vi "电流判定.vi"(7 "Result":refnum<vi>, 9 "索引":u8, 10 "判定参数":T1, 11 "XY曲线":cluster{"X":dbl[], "Y":dbl[]}[](array[cluster])) -> (3 "OK？":bool)   [LabVIEW 2020]
panel:
  out "目标5逆向输入扭矩":dbl
  out "目标5正向输入扭矩":dbl
  out "目标 5":dbl
  out "目标4逆向输入扭矩":dbl
  out "目标4正向输入扭矩":dbl
  out "目标 4":dbl
  out "目标3逆向输入扭矩":dbl
  out "目标3正向输入扭矩":dbl
  out "目标 3":dbl
  out "目标2逆向输入扭矩":dbl
  out "目标2正向输入扭矩":dbl
  out "目标 2":dbl
  out "目标1正向输入扭矩":dbl
  out "目标1逆向输入扭矩":dbl
  out "目标 1":dbl
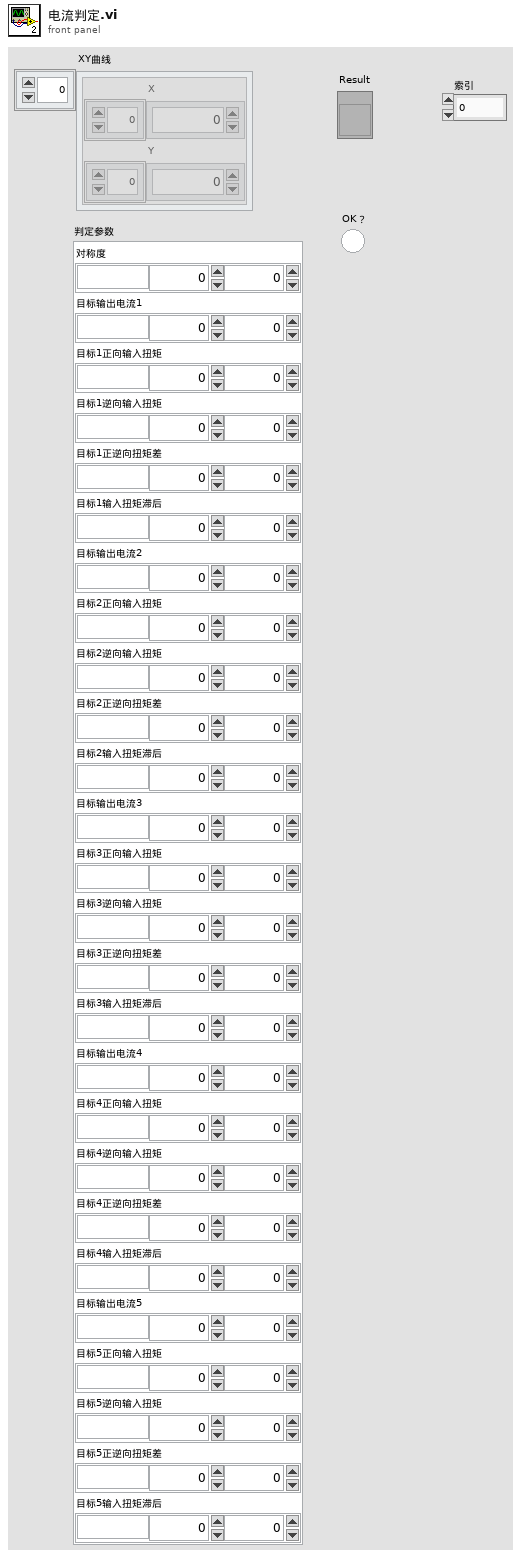
[diagram p1: front panel]
types:
  T1 = cluster{"对称度":cluster{"单位":string, "下限":dbl, "上限":dbl}, "目标输出电流1":cluster{"单位":string, "下限":dbl, "上限":dbl}, "目标1正向输入扭矩":cluster{"单位":string, "下限":dbl, "上限":dbl}, "目标1逆向输入扭矩":cluster{"单位":string, "下限":dbl, "上限":dbl}, "目标1正逆向扭矩差":cluster{"单位":string, "下限":dbl, "上限":dbl}, "目标1输入扭矩滞后":cluster{"单位":string, "下限":dbl, "上限":dbl}, "目标输出电流2":cluster{"单位":string, "下限":dbl, "上限":dbl}, "目标2正向输入扭矩":cluster{"单位":string, "下限":dbl, "上限":dbl}, "目标2逆向输入扭矩":cluster{"单位":string, "下限":dbl, "上限":dbl}, "目标2正逆向扭矩差":cluster{"单位":string, "下限":dbl, "上限":dbl}, "目标2输入扭矩滞后":cluster{"单位":string, "下限":dbl, "上限":dbl}, "目标输出电流3":cluster{"单位":string, "下限":dbl, "上限":dbl}, "目标3正向输入扭矩":cluster{"单位":string, "下限":dbl, "上限":dbl}, "目标3逆向输入扭矩":cluster{"单位":string, "下限":dbl, "上限":dbl}, "目标3正逆向扭矩差":cluster{"单位":string, "下限":dbl, "上限":dbl}, "目标3输入扭矩滞后":cluster{"单位":string, "下限":dbl, "上限":dbl}, "目标输出电流4":cluster{"单位":string, "下限":dbl, "上限":dbl}, "目标4正向输入扭矩":cluster{"单位":string, "下限":dbl, "上限":dbl}, "目标4逆向输入扭矩":cluster{"单位":string, "下限":dbl, "上限":dbl}, "目标4正逆向扭矩差":cluster{"单位":string, "下限":dbl, "上限":dbl}, "目标4输入扭矩滞后":cluster{"单位":string, "下限":dbl, "上限":dbl}, "目标输出电流5":cluster{"单位":string, "下限":dbl, "上限":dbl}, "目标5正向输入扭矩":cluster{"单位":string, "下限":dbl, "上限":dbl}, "目标5逆向输入扭矩":cluster{"单位":string, "下限":dbl, "上限":dbl}, "目标5正逆向扭矩差":cluster{"单位":string, "下限":dbl, "上限":dbl}, "目标5输入扭矩滞后":cluster{"单位":string, "下限":dbl, "上限":dbl}}
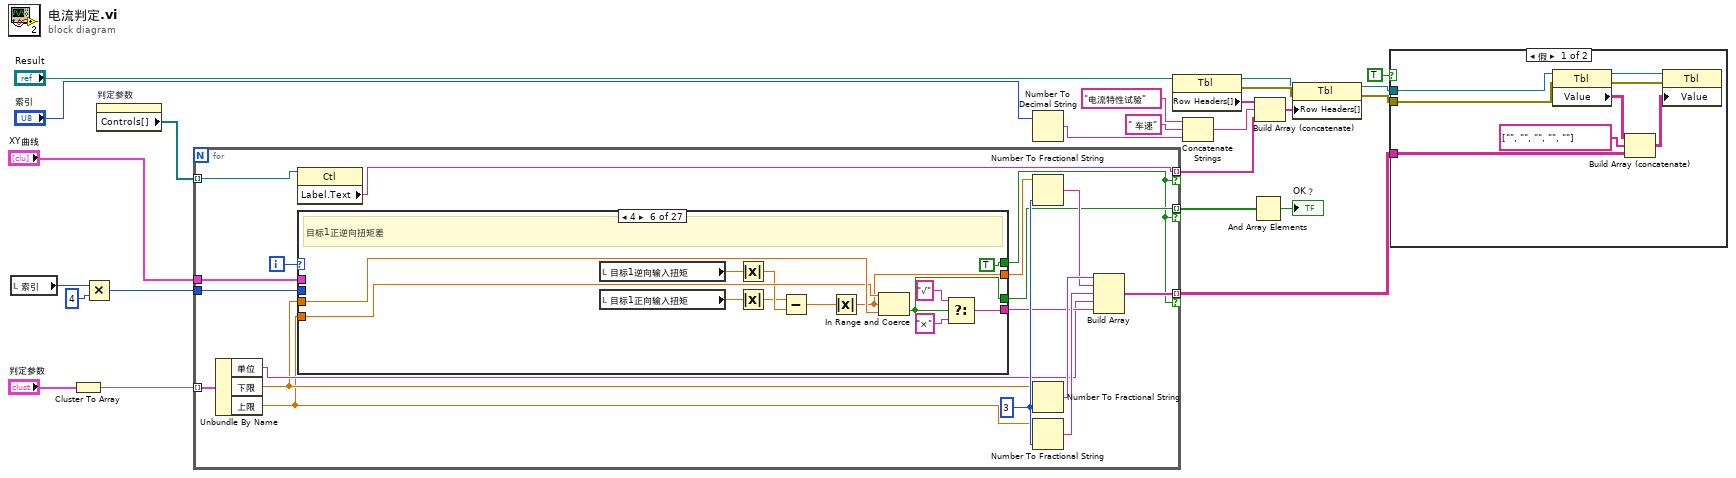
[diagram p0: block diagram]
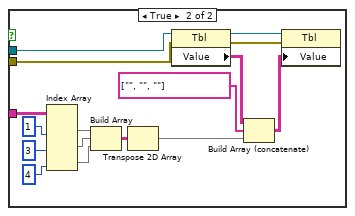
[diagram p2: hidden frame]
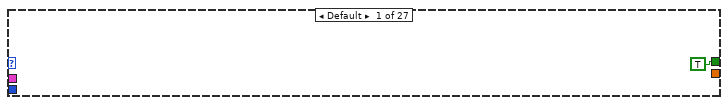
[diagram p3: hidden frame]
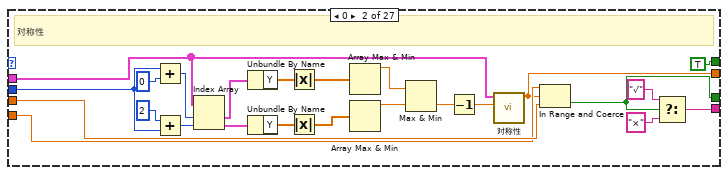
[diagram p4: hidden frame]
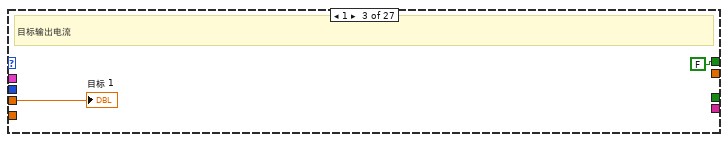
[diagram p5: hidden frame]
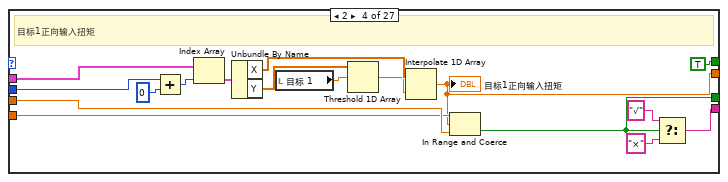
[diagram p6: hidden frame]
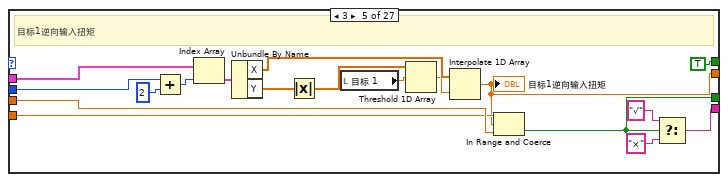
[diagram p7: hidden frame]
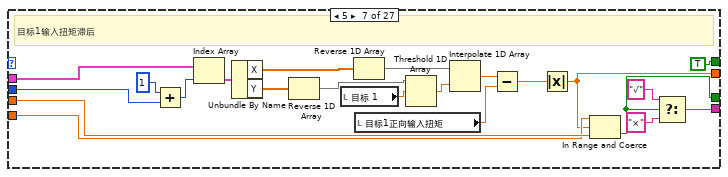
[diagram p8: hidden frame]
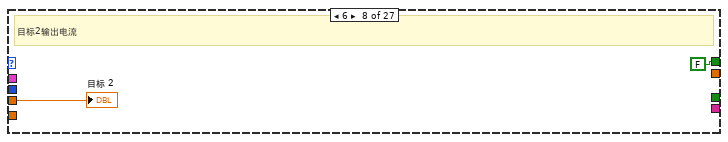
[diagram p9: hidden frame]
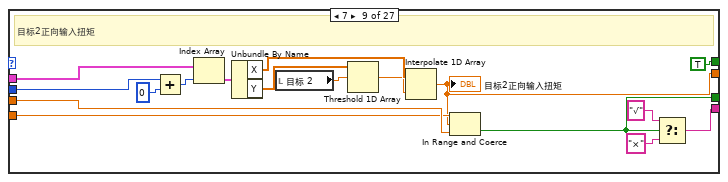
[diagram p10: hidden frame]
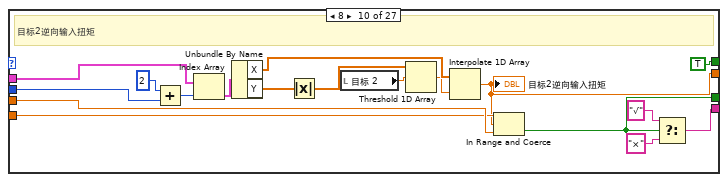
[diagram p11: hidden frame]
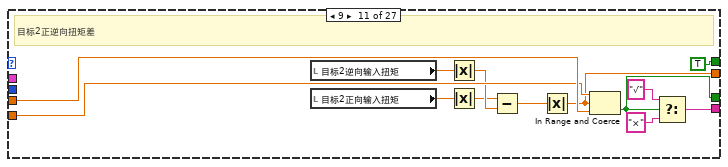
[diagram p12: hidden frame]
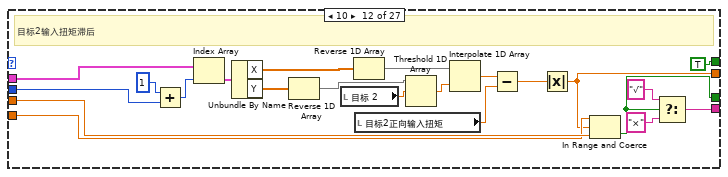
[diagram p13: hidden frame]
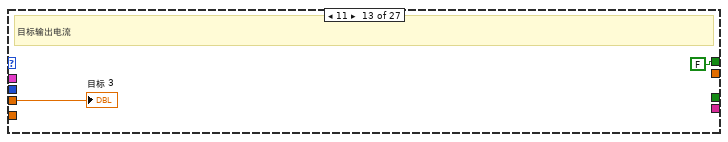
[diagram p14: hidden frame]
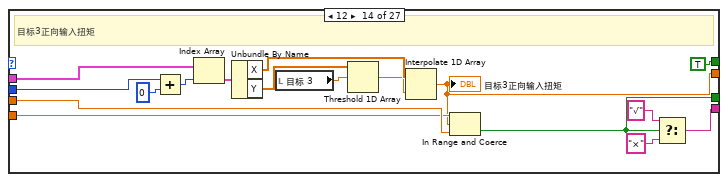
[diagram p15: hidden frame]
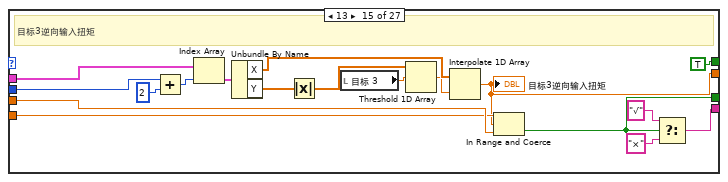
[diagram p16: hidden frame]
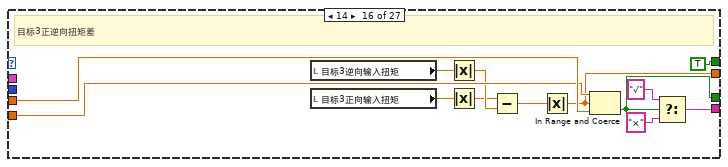
[diagram p17: hidden frame]
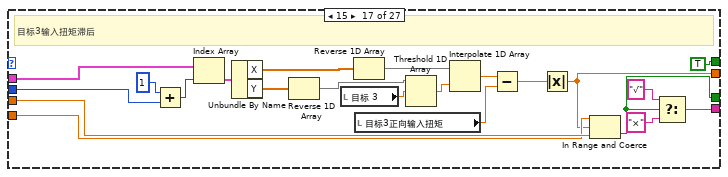
[diagram p18: hidden frame]
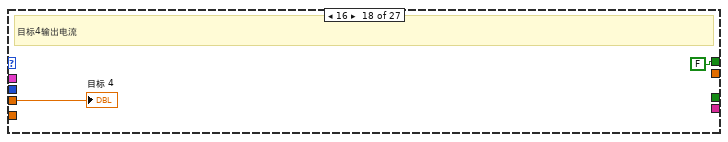
[diagram p19: hidden frame]
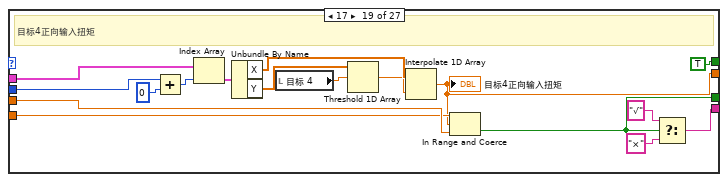
[diagram p20: hidden frame]
diagram:
  n1 = local read "索引"() -> (w3:u8)
  n2 = Cluster To Array(cluster="判定参数") -> (array=w24:cluster{"单位":string, "下限":dbl, "上限":dbl}[])
  n3 = Multiply(x=w3, y=u8 4) -> (x*y=w1:u8)
  n4 = property on="判定参数" class="Clust (严格)"() -> ("Controls[]"=w10:refnum<vi>[])  [unwired: 2 in, 2 out]
  n5 = for {
    tunnel: w24 -> [w42] mode=indexing
    tunnel: w10 -> [w40] mode=indexing
    tunnel: "XY曲线" -> [w38]
    tunnel: [w32] -> w22 mode=indexing if=w26
    tunnel: [w28] -> w12 mode=indexing if=w26
    tunnel: [w27] -> w15 mode=indexing if=w26
    tunnel: w1 -> [w25]
    i -> [w41]
    w37 = i16 3 ("精度(6)")
    n6 = Unbundle By Name(w42) -> ("单位"=w31:string, "下限"=w30:dbl, "上限"=w29:dbl)
    n7 = property class="Ctl"(reference=w40) -> ("Label.Text"=w27:string)  [unwired: 1 in, 2 out]
    n8 = case shown="4" w41 {
      tunnel: [_ w52 _ w72 w91 w107 w121 _ w144 w163 w179 w193 _ w216 w235 w251 w265 _ w288 w307 w323 w337 _ w360 w379 w395 w409] -> w39
      tunnel: w38 -> [_ w56 _ w79 w97 _ w133 _ w151 w169 _ w205 _ w223 w241 _ w277 _ w295 w313 _ w349 _ w367 w385 _ w421]
      tunnel: [_ w61 _ w84 w102 w115 w122 _ w156 w174 w187 w194 _ w228 w246 w259 w266 _ w300 w318 w331 w338 _ w372 w390 w403 w410] -> w33
      tunnel: [_ w60 _ w83 w101 w114 w123 _ w155 w173 w186 w195 _ w227 w245 w258 w267 _ w299 w317 w330 w339 _ w371 w389 w402 w411] -> w32
      tunnel: w30 -> [_ w59 w68 w82 w100 w113 w127 w140 w154 w172 w185 w199 w212 w226 w244 w257 w271 w284 w298 w316 w329 w343 w356 w370 w388 w401 w415]
      tunnel: w29 -> [_ w58 _ w81 w99 w112 w126 _ w153 w171 w184 w198 _ w225 w243 w256 w270 _ w297 w315 w328 w342 _ w369 w387 w400 w414]
      tunnel: [TRUE TRUE FALSE TRUE TRUE TRUE TRUE FALSE TRUE TRUE TRUE TRUE FALSE TRUE TRUE TRUE TRUE FALSE TRUE TRUE TRUE TRUE FALSE TRUE TRUE TRUE TRUE] -> w26
      tunnel: w25 -> [_ w44 _ w70 w87 _ w118 _ w142 w159 _ w190 _ w214 w231 _ w262 _ w286 w303 _ w334 _ w358 w375 _ w406]
      frame Default {
      }
      frame 0 {
        # "对称性"
        n9 = Add(x=w44, y=0 ("索引")) -> (x+y=w46:i32)
        n10 = Add(x=2 ("索引"), y=w44) -> (x+y=w45:i32)
        n11 = Index Array(array=w56, index #1=w46, index #2=w45) -> (element #1=w65:cluster{"X":dbl[], "Y":dbl[]}, element #2=w64:cluster{"X":dbl[], "Y":dbl[]})
        n12 = Unbundle By Name(w65) -> ("Y"=w55:dbl[])
        n13 = Unbundle By Name(w64) -> ("Y"=w54:dbl[])
        n14 = Absolute Value(x=w55) -> (abs(x)=w51:dbl[])
        n15 = Absolute Value(x=w54) -> (abs(x)=w50:dbl[])
        n16 = Array Max & Min(array=w51) -> (max value=w49:dbl)  [unwired: 3 out]
        n17 = Array Max & Min(array=w50) -> (max value=w48:dbl)  [unwired: 3 out]
        n18 = Max & Min(x=w49, y=w48) -> (min(x,y)=w53:dbl)  [unwired: 1 out]
        n19 = Decrement(x=w53) -> (x-1=w47:dbl)
        n20 = call "对称性.vi"("定点"=w47, "XY图"=w56) -> ("对称性"=w52:dbl)  [unwired: 9 in]
        n21 = In Range and Coerce(upper limit=w58, x=w52, lower limit=w59) -> (In Range?=w60:bool)  [unwired: 1 out]
        n22 = Select(t="√", s=w60, f="×") -> (s? t:f=w61:string)
      }
      frame 1 {
        # "目标输出电流"
        "目标 1" <- w68
      }
      frame 2 {
        # "目标1正向输入扭矩"
        n23 = Add(x=w70, y=0 ("索引")) -> (x+y=w71:i32)
        n24 = Index Array(array=w79, index=w71) -> (element=w78:cluster{"X":dbl[], "Y":dbl[]})
        n25 = Unbundle By Name(w78) -> ("X"=w75:dbl[], "Y"=w77:dbl[])
        n26 = local read "目标 1"() -> (w76:dbl)
        n27 = Threshold 1D Array(2:w76, 3:w77) -> (0:w74:dbl)  [unwired: 1 in]
        n28 = Interpolate 1D Array(1:w74, 2:w75) -> (0:w72:dbl)
        "目标1正向输入扭矩" <- w72
        n29 = In Range and Coerce(upper limit=w81, x=w72, lower limit=w82) -> (In Range?=w83:bool)  [unwired: 1 out]
        n30 = Select(t="√", s=w83, f="×") -> (s? t:f=w84:string)
      }
      frame 3 {
        # "目标1逆向输入扭矩"
        n31 = Add(x=w87, y=2 ("索引")) -> (x+y=w88:i32)
        n32 = Index Array(array=w97, index=w88) -> (element=w96:cluster{"X":dbl[], "Y":dbl[]})
        n33 = Unbundle By Name(w96) -> ("X"=w93:dbl[], "Y"=w95:dbl[])
        n34 = Absolute Value(x=w95) -> (abs(x)=w89:dbl[])
        n35 = local read "目标 1"() -> (w94:dbl)
        n36 = Threshold 1D Array(2:w94, 3:w89) -> (0:w92:dbl)  [unwired: 1 in]
        n37 = Interpolate 1D Array(1:w92, 2:w93) -> (0:w91:dbl)
        "目标1逆向输入扭矩" <- w91
        n38 = In Range and Coerce(upper limit=w99, x=w91, lower limit=w100) -> (In Range?=w101:bool)  [unwired: 1 out]
        n39 = Select(t="√", s=w101, f="×") -> (s? t:f=w102:string)
      }
      frame 4 {
        # "目标1正逆向扭矩差"
        n40 = local read "目标1逆向输入扭矩"() -> (w109:dbl)
        n41 = local read "目标1正向输入扭矩"() -> (w110:dbl)
        n42 = Absolute Value(x=w109) -> (abs(x)=w106:dbl)
        n43 = Absolute Value(x=w110) -> (abs(x)=w105:dbl)
        n44 = Subtract(x=w105, y=w106) -> (x-y=w108:dbl)
        n45 = Absolute Value(x=w108) -> (abs(x)=w107:dbl)
        n46 = In Range and Coerce(upper limit=w112, x=w107, lower limit=w113) -> (In Range?=w114:bool)  [unwired: 1 out]
        n47 = Select(t="√", s=w114, f="×") -> (s? t:f=w115:string)
      }
      frame 5 {
        # "目标1输入扭矩滞后"
        n48 = Add(x=1 ("索引"), y=w118) -> (x+y=w119:i32)
        n49 = Index Array(array=w133, index=w119) -> (element=w139:cluster{"X":dbl[], "Y":dbl[]})
        n50 = Unbundle By Name(w139) -> ("X"=w136:dbl[], "Y"=w138:dbl[])
        n51 = Reverse 1D Array(array=w138) -> (reversed array=w132:dbl[])
        n52 = local read "目标 1"() -> (w137:dbl)
        n53 = Reverse 1D Array(array=w136) -> (reversed array=w131:dbl[])
        n54 = local read "目标1正向输入扭矩"() -> (w129:dbl)
        n55 = Threshold 1D Array(2:w137, 3:w132) -> (0:w135:dbl)  [unwired: 1 in]
        n56 = Interpolate 1D Array(1:w135, 2:w131) -> (0:w130:dbl)
        n57 = Subtract(x=w130, y=w129) -> (x-y=w128:dbl)
        n58 = Absolute Value(x=w128) -> (abs(x)=w121:dbl)
        n59 = In Range and Coerce(upper limit=w126, x=w121, lower limit=w127) -> (In Range?=w123:bool)  [unwired: 1 out]
        n60 = Select(t="√", s=w123, f="×") -> (s? t:f=w122:string)
      }
      frame 6 {
        # "目标2输出电流"
        "目标 2" <- w140
      }
      frame 7 {
        # "目标2正向输入扭矩"
        n61 = Add(x=w142, y=0 ("索引")) -> (x+y=w143:i32)
        n62 = Index Array(array=w151, index=w143) -> (element=w150:cluster{"X":dbl[], "Y":dbl[]})
        n63 = Unbundle By Name(w150) -> ("X"=w147:dbl[], "Y"=w149:dbl[])
        n64 = local read "目标 2"() -> (w148:dbl)
        n65 = Threshold 1D Array(2:w148, 3:w149) -> (0:w146:dbl)  [unwired: 1 in]
        n66 = Interpolate 1D Array(1:w146, 2:w147) -> (0:w144:dbl)
        "目标2正向输入扭矩" <- w144
        n67 = In Range and Coerce(upper limit=w153, x=w144, lower limit=w154) -> (In Range?=w155:bool)  [unwired: 1 out]
        n68 = Select(t="√", s=w155, f="×") -> (s? t:f=w156:string)
      }
      frame 8 {
        # "目标2逆向输入扭矩"
        n69 = Add(x=2 ("索引"), y=w159) -> (x+y=w160:i32)
        n70 = Index Array(array=w169, index=w160) -> (element=w168:cluster{"X":dbl[], "Y":dbl[]})
        n71 = Unbundle By Name(w168) -> ("X"=w165:dbl[], "Y"=w167:dbl[])
        n72 = Absolute Value(x=w167) -> (abs(x)=w161:dbl[])
        n73 = local read "目标 2"() -> (w166:dbl)
        n74 = Threshold 1D Array(2:w166, 3:w161) -> (0:w164:dbl)  [unwired: 1 in]
        n75 = Interpolate 1D Array(1:w164, 2:w165) -> (0:w163:dbl)
        "目标2逆向输入扭矩" <- w163
        n76 = In Range and Coerce(upper limit=w171, x=w163, lower limit=w172) -> (In Range?=w173:bool)  [unwired: 1 out]
        n77 = Select(t="√", s=w173, f="×") -> (s? t:f=w174:string)
      }
      frame 9 {
        # "目标2正逆向扭矩差"
        n78 = local read "目标2逆向输入扭矩"() -> (w181:dbl)
        n79 = local read "目标2正向输入扭矩"() -> (w182:dbl)
        n80 = Absolute Value(x=w181) -> (abs(x)=w178:dbl)
        n81 = Absolute Value(x=w182) -> (abs(x)=w177:dbl)
        n82 = Subtract(x=w177, y=w178) -> (x-y=w180:dbl)
        n83 = Absolute Value(x=w180) -> (abs(x)=w179:dbl)
        n84 = In Range and Coerce(upper limit=w184, x=w179, lower limit=w185) -> (In Range?=w186:bool)  [unwired: 1 out]
        n85 = Select(t="√", s=w186, f="×") -> (s? t:f=w187:string)
      }
      frame 10 {
        # "目标2输入扭矩滞后"
        n86 = Add(x=1 ("索引"), y=w190) -> (x+y=w191:i32)
        n87 = Index Array(array=w205, index=w191) -> (element=w211:cluster{"X":dbl[], "Y":dbl[]})
        n88 = Unbundle By Name(w211) -> ("X"=w208:dbl[], "Y"=w210:dbl[])
        n89 = Reverse 1D Array(array=w210) -> (reversed array=w204:dbl[])
        n90 = local read "目标 2"() -> (w209:dbl)
        n91 = Reverse 1D Array(array=w208) -> (reversed array=w203:dbl[])
        n92 = local read "目标2正向输入扭矩"() -> (w201:dbl)
        n93 = Threshold 1D Array(2:w209, 3:w204) -> (0:w207:dbl)  [unwired: 1 in]
        n94 = Interpolate 1D Array(1:w207, 2:w203) -> (0:w202:dbl)
        n95 = Subtract(x=w202, y=w201) -> (x-y=w200:dbl)
        n96 = Absolute Value(x=w200) -> (abs(x)=w193:dbl)
        n97 = In Range and Coerce(upper limit=w198, x=w193, lower limit=w199) -> (In Range?=w195:bool)  [unwired: 1 out]
        n98 = Select(t="√", s=w195, f="×") -> (s? t:f=w194:string)
      }
      frame 11 {
        # "目标输出电流"
        "目标 3" <- w212
      }
      frame 12 {
        # "目标3正向输入扭矩"
        n99 = Add(x=w214, y=0 ("索引")) -> (x+y=w215:i32)
        n100 = Index Array(array=w223, index=w215) -> (element=w222:cluster{"X":dbl[], "Y":dbl[]})
        n101 = Unbundle By Name(w222) -> ("X"=w219:dbl[], "Y"=w221:dbl[])
        n102 = local read "目标 3"() -> (w220:dbl)
        n103 = Threshold 1D Array(2:w220, 3:w221) -> (0:w218:dbl)  [unwired: 1 in]
        n104 = Interpolate 1D Array(1:w218, 2:w219) -> (0:w216:dbl)
        "目标3正向输入扭矩" <- w216
        n105 = In Range and Coerce(upper limit=w225, x=w216, lower limit=w226) -> (In Range?=w227:bool)  [unwired: 1 out]
        n106 = Select(t="√", s=w227, f="×") -> (s? t:f=w228:string)
      }
      frame 13 {
        # "目标3逆向输入扭矩"
        n107 = Add(x=w231, y=2 ("索引")) -> (x+y=w232:i32)
        n108 = Index Array(array=w241, index=w232) -> (element=w240:cluster{"X":dbl[], "Y":dbl[]})
        n109 = Unbundle By Name(w240) -> ("X"=w237:dbl[], "Y"=w239:dbl[])
        n110 = Absolute Value(x=w239) -> (abs(x)=w233:dbl[])
        n111 = local read "目标 3"() -> (w238:dbl)
        n112 = Threshold 1D Array(2:w238, 3:w233) -> (0:w236:dbl)  [unwired: 1 in]
        n113 = Interpolate 1D Array(1:w236, 2:w237) -> (0:w235:dbl)
        "目标3逆向输入扭矩" <- w235
        n114 = In Range and Coerce(upper limit=w243, x=w235, lower limit=w244) -> (In Range?=w245:bool)  [unwired: 1 out]
        n115 = Select(t="√", s=w245, f="×") -> (s? t:f=w246:string)
      }
      frame 14 {
        # "目标3正逆向扭矩差"
        n116 = local read "目标3逆向输入扭矩"() -> (w253:dbl)
        n117 = local read "目标3正向输入扭矩"() -> (w254:dbl)
        n118 = Absolute Value(x=w253) -> (abs(x)=w250:dbl)
        n119 = Absolute Value(x=w254) -> (abs(x)=w249:dbl)
        n120 = Subtract(x=w249, y=w250) -> (x-y=w252:dbl)
        n121 = Absolute Value(x=w252) -> (abs(x)=w251:dbl)
        n122 = In Range and Coerce(upper limit=w256, x=w251, lower limit=w257) -> (In Range?=w258:bool)  [unwired: 1 out]
        n123 = Select(t="√", s=w258, f="×") -> (s? t:f=w259:string)
      }
      frame 15 {
        # "目标3输入扭矩滞后"
        n124 = Add(x=1 ("索引"), y=w262) -> (x+y=w263:i32)
        n125 = Index Array(array=w277, index=w263) -> (element=w283:cluster{"X":dbl[], "Y":dbl[]})
        n126 = Unbundle By Name(w283) -> ("X"=w280:dbl[], "Y"=w282:dbl[])
        n127 = Reverse 1D Array(array=w282) -> (reversed array=w276:dbl[])
        n128 = local read "目标 3"() -> (w281:dbl)
        n129 = Reverse 1D Array(array=w280) -> (reversed array=w275:dbl[])
        n130 = local read "目标3正向输入扭矩"() -> (w273:dbl)
        n131 = Threshold 1D Array(2:w281, 3:w276) -> (0:w279:dbl)  [unwired: 1 in]
        n132 = Interpolate 1D Array(1:w279, 2:w275) -> (0:w274:dbl)
        n133 = Subtract(x=w274, y=w273) -> (x-y=w272:dbl)
        n134 = Absolute Value(x=w272) -> (abs(x)=w265:dbl)
        n135 = In Range and Coerce(upper limit=w270, x=w265, lower limit=w271) -> (In Range?=w267:bool)  [unwired: 1 out]
        n136 = Select(t="√", s=w267, f="×") -> (s? t:f=w266:string)
      }
      frame 16 {
        # "目标4输出电流"
        "目标 4" <- w284
      }
      frame 17 {
        # "目标4正向输入扭矩"
        n137 = Add(x=w286, y=0 ("索引")) -> (x+y=w287:i32)
        n138 = Index Array(array=w295, index=w287) -> (element=w294:cluster{"X":dbl[], "Y":dbl[]})
        n139 = Unbundle By Name(w294) -> ("X"=w291:dbl[], "Y"=w293:dbl[])
        n140 = local read "目标 4"() -> (w292:dbl)
        n141 = Threshold 1D Array(2:w292, 3:w293) -> (0:w290:dbl)  [unwired: 1 in]
        n142 = Interpolate 1D Array(1:w290, 2:w291) -> (0:w288:dbl)
        "目标4正向输入扭矩" <- w288
        n143 = In Range and Coerce(upper limit=w297, x=w288, lower limit=w298) -> (In Range?=w299:bool)  [unwired: 1 out]
        n144 = Select(t="√", s=w299, f="×") -> (s? t:f=w300:string)
      }
      frame 18 {
        # "目标4逆向输入扭矩"
        n145 = Add(x=w303, y=2 ("索引")) -> (x+y=w304:i32)
        n146 = Index Array(array=w313, index=w304) -> (element=w312:cluster{"X":dbl[], "Y":dbl[]})
        n147 = Unbundle By Name(w312) -> ("X"=w309:dbl[], "Y"=w311:dbl[])
        n148 = Absolute Value(x=w311) -> (abs(x)=w305:dbl[])
        n149 = local read "目标 4"() -> (w310:dbl)
        n150 = Threshold 1D Array(2:w310, 3:w305) -> (0:w308:dbl)  [unwired: 1 in]
        n151 = Interpolate 1D Array(1:w308, 2:w309) -> (0:w307:dbl)
        "目标4逆向输入扭矩" <- w307
        n152 = In Range and Coerce(upper limit=w315, x=w307, lower limit=w316) -> (In Range?=w317:bool)  [unwired: 1 out]
        n153 = Select(t="√", s=w317, f="×") -> (s? t:f=w318:string)
      }
      frame 19 {
        # "目标4正逆向扭矩差"
        n154 = local read "目标4逆向输入扭矩"() -> (w325:dbl)
        n155 = local read "目标4正向输入扭矩"() -> (w326:dbl)
        n156 = Absolute Value(x=w325) -> (abs(x)=w322:dbl)
        n157 = Absolute Value(x=w326) -> (abs(x)=w321:dbl)
        n158 = Subtract(x=w321, y=w322) -> (x-y=w324:dbl)
        n159 = Absolute Value(x=w324) -> (abs(x)=w323:dbl)
        n160 = In Range and Coerce(upper limit=w328, x=w323, lower limit=w329) -> (In Range?=w330:bool)  [unwired: 1 out]
        n161 = Select(t="√", s=w330, f="×") -> (s? t:f=w331:string)
      }
      frame 20 {
        # "目标4输入扭矩滞后"
        n162 = Add(x=w334, y=1 ("索引")) -> (x+y=w335:i32)
        n163 = Index Array(array=w349, index=w335) -> (element=w355:cluster{"X":dbl[], "Y":dbl[]})
        n164 = Unbundle By Name(w355) -> ("X"=w352:dbl[], "Y"=w354:dbl[])
        n165 = Reverse 1D Array(array=w354) -> (reversed array=w348:dbl[])
        n166 = local read "目标 4"() -> (w353:dbl)
        n167 = Reverse 1D Array(array=w352) -> (reversed array=w347:dbl[])
        n168 = local read "目标4正向输入扭矩"() -> (w345:dbl)
        n169 = Threshold 1D Array(2:w353, 3:w348) -> (0:w351:dbl)  [unwired: 1 in]
        n170 = Interpolate 1D Array(1:w351, 2:w347) -> (0:w346:dbl)
        n171 = Subtract(x=w346, y=w345) -> (x-y=w344:dbl)
        n172 = Absolute Value(x=w344) -> (abs(x)=w337:dbl)
        n173 = In Range and Coerce(upper limit=w342, x=w337, lower limit=w343) -> (In Range?=w339:bool)  [unwired: 1 out]
        n174 = Select(t="√", s=w339, f="×") -> (s? t:f=w338:string)
      }
      frame 21 {
        # "目标5输出电流"
        "目标 5" <- w356
      }
      frame 22 {
        # "目标5正向输入扭矩"
        n175 = Add(x=0 ("索引"), y=w358) -> (x+y=w359:i32)
        n176 = Index Array(array=w367, index=w359) -> (element=w366:cluster{"X":dbl[], "Y":dbl[]})
        n177 = Unbundle By Name(w366) -> ("X"=w363:dbl[], "Y"=w365:dbl[])
        n178 = local read "目标 5"() -> (w364:dbl)
        n179 = Threshold 1D Array(2:w364, 3:w365) -> (0:w362:dbl)  [unwired: 1 in]
        n180 = Interpolate 1D Array(1:w362, 2:w363) -> (0:w360:dbl)
        "目标5正向输入扭矩" <- w360
        n181 = In Range and Coerce(upper limit=w369, x=w360, lower limit=w370) -> (In Range?=w371:bool)  [unwired: 1 out]
        n182 = Select(t="√", s=w371, f="×") -> (s? t:f=w372:string)
      }
      frame 23 {
        # "目标5逆向输入扭矩"
        n183 = Add(x=2 ("索引"), y=w375) -> (x+y=w376:i32)
        n184 = Index Array(array=w385, index=w376) -> (element=w384:cluster{"X":dbl[], "Y":dbl[]})
        n185 = Unbundle By Name(w384) -> ("X"=w381:dbl[], "Y"=w383:dbl[])
        n186 = Absolute Value(x=w383) -> (abs(x)=w377:dbl[])
        n187 = local read "目标 5"() -> (w382:dbl)
        n188 = Threshold 1D Array(2:w382, 3:w377) -> (0:w380:dbl)  [unwired: 1 in]
        n189 = Interpolate 1D Array(1:w380, 2:w381) -> (0:w379:dbl)
        "目标5逆向输入扭矩" <- w379
        n190 = In Range and Coerce(upper limit=w387, x=w379, lower limit=w388) -> (In Range?=w389:bool)  [unwired: 1 out]
        n191 = Select(t="√", s=w389, f="×") -> (s? t:f=w390:string)
      }
      frame 24 {
        # "目标5正逆向扭矩差"
        n192 = local read "目标5逆向输入扭矩"() -> (w397:dbl)
        n193 = local read "目标5正向输入扭矩"() -> (w398:dbl)
        n194 = Absolute Value(x=w397) -> (abs(x)=w394:dbl)
        n195 = Absolute Value(x=w398) -> (abs(x)=w393:dbl)
        n196 = Subtract(x=w393, y=w394) -> (x-y=w396:dbl)
        n197 = Absolute Value(x=w396) -> (abs(x)=w395:dbl)
        n198 = In Range and Coerce(upper limit=w400, x=w395, lower limit=w401) -> (In Range?=w402:bool)  [unwired: 1 out]
        n199 = Select(t="√", s=w402, f="×") -> (s? t:f=w403:string)
      }
      frame 25 {
        # "目标5输入扭矩滞后"
        n200 = Add(x=1 ("索引"), y=w406) -> (x+y=w407:i32)
        n201 = Index Array(array=w421, index=w407) -> (element=w427:cluster{"X":dbl[], "Y":dbl[]})
        n202 = Unbundle By Name(w427) -> ("X"=w424:dbl[], "Y"=w426:dbl[])
        n203 = Reverse 1D Array(array=w426) -> (reversed array=w420:dbl[])
        n204 = local read "目标 5"() -> (w425:dbl)
        n205 = Reverse 1D Array(array=w424) -> (reversed array=w419:dbl[])
        n206 = local read "目标5正向输入扭矩"() -> (w417:dbl)
        n207 = Threshold 1D Array(2:w425, 3:w420) -> (0:w423:dbl)  [unwired: 1 in]
        n208 = Interpolate 1D Array(1:w423, 2:w419) -> (0:w418:dbl)
        n209 = Subtract(x=w418, y=w417) -> (x-y=w416:dbl)
        n210 = Absolute Value(x=w416) -> (abs(x)=w409:dbl)
        n211 = In Range and Coerce(upper limit=w414, x=w409, lower limit=w415) -> (In Range?=w411:bool)  [unwired: 1 out]
        n212 = Select(t="√", s=w411, f="×") -> (s? t:f=w410:string)
      }
    }
    n213 = Number To Fractional String(number=w39, precision (6)=w37) -> (F-format string=w35:string)  [unwired: 2 in]
    n214 = Number To Fractional String(number=w30, precision (6)=w37) -> (F-format string=w36:string)  [unwired: 2 in]
    n215 = Number To Fractional String(number=w29, precision (6)=w37) -> (F-format string=w34:string)  [unwired: 2 in]
    n216 = Build Array(w36, w35, w34, w31, w33) -> (w28:string[])
  }
  n217 = Number To Decimal String(number="索引") -> (decimal integer string=w7:string)  [unwired: 1 in]
  n218 = property class="Tbl"(reference="Result") -> (reference out=w17:refnum<vi>, error out=w20:errorcluster, "Row Headers[]"=w13:string[])  [unwired: 1 in]
  n219 = Concatenate Strings("电流特性试验" ("Label.Text"), " 车速" ("字符串"), w7) -> (w4:string)
  n220 = And Array Elements(Boolean array=w22) -> (logical AND=→"OK？":bool)
  n221 = Build Array (concatenate)(w13, w4, w15) -> (w16:string[])
  n222 = property class="Tbl"(reference=w17, error in=w20, "Row Headers[]"=w16) -> (reference out=w18:refnum<vi>, error out=w19:errorcluster)
  n223 = case shown="假" TRUE {
    tunnel: w19 -> [w433 w449]
    tunnel: w18 -> [w430 w446]
    tunnel: w12 -> [w429 w437]
    frame False {
      n224 = property class="Tbl"(reference=w430, error in=w433) -> (reference out=w431:refnum<vi>, error out=w432:errorcluster, "Value"=w434:string[][])
      n225 = Build Array (concatenate)(w434, string[] ["", "", "", "", ""], w429) -> (w435:string[][])
      n226 = property class="Tbl"(reference=w431, error in=w432, "Value"=w435) -> ()  [unwired: 2 out]
    }
    frame True {
      n227 = Index Array(array=w437, index (col) #1=1 ("禁用的索引 (列)"), index (col) #2=3 ("索引 (列)"), index (col) #3=4 ("索引 (列)")) -> (element #1=w441:string[], element #2=w440:string[], element #3=w439:string[])  [unwired: 3 in]
      n228 = Build Array(w441, w440, w439) -> (w438:string[][])
      n229 = Transpose 2D Array(2D array=w438) -> (transposed array=w436:string[][])
      n230 = property class="Tbl"(reference=w446, error in=w449) -> (reference out=w447:refnum<vi>, error out=w448:errorcluster, "Value"=w450:string[][])
      n231 = Build Array (concatenate)(w450, string[] ["", "", ""], w436) -> (w451:string[][])
      n232 = property class="Tbl"(reference=w447, error in=w448, "Value"=w451) -> ()  [unwired: 2 out]
    }
  }
